vi "Shoot.vi"(2 "Stack Loaded?":bool=TRUE, 3 "Ready 2 Shoot?":bool=TRUE, 4 "Fire":bool=TRUE, 5 "Override":bool=TRUE) -> (0 "Le Fire at Will?":bool, 1 "Top":dbl)   [LabVIEW 2011]
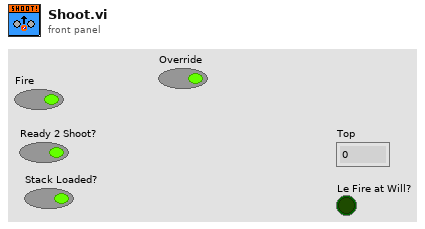
[diagram p1: front panel]
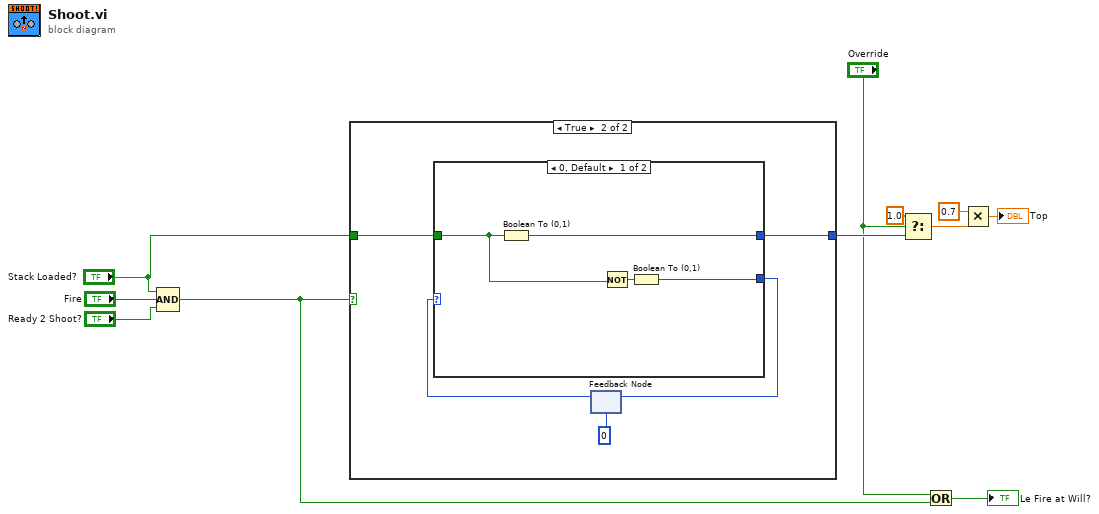
[diagram p0: block diagram]
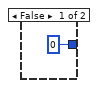
[diagram p2: hidden frame]
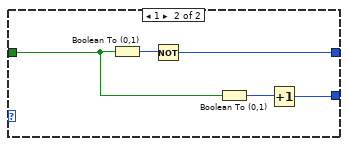
[diagram p3: hidden frame]
diagram:
  n1 = Compound Arithmetic op=AND("Stack Loaded?", "Fire", "Ready 2 Shoot?") -> (w6:bool)
  n2 = case shown="True" w6 {
    tunnel: "Stack Loaded?" -> [_ w14]
    tunnel: [i16 0 w13] -> w8
    frame False {
    }
    frame True {
      n3 = feedback #1(0) -> (w16:i32)
      n4 = case shown="0, Default" w16 {
        tunnel: [w18 w22] -> w17
        tunnel: w14 -> [w19 w24]
        tunnel: [w21 w25] -> w13
        frame 0, Default {
          n5 = Boolean To (0,1)(Boolean=w19) -> (0, 1=w21:i16)
          n6 = Not(x=w19) -> (.not. x?=w20:bool)
          n7 = Boolean To (0,1)(Boolean=w20) -> (0, 1=w18:i16)
        }
        frame 1 {
          n8 = Boolean To (0,1)(Boolean=w24) -> (0, 1=w26:i16)
          n9 = Not(x=w26) -> (.not. x?=w25:i16)
          n10 = Boolean To (0,1)(Boolean=w24) -> (0, 1=w23:i16)
          n11 = Increment(x=w23) -> (x+1=w22:i16)
        }
      }
      n12 = feedback-in #1(w17) -> ()
    }
  }
  n13 = Select(t=1.0 ("x"), s="Override", f=w8) -> (s? t:f=w7:dbl)
  n14 = Or(x="Override", y=w6) -> (x .or. y?=→"Le Fire at Will?":bool)
  n15 = Multiply(x=0.7, y=w7) -> (x*y=→"Top":dbl)
